vi "fgt set log output mode.vi"(8 "error in (no error)":errorcluster, 9 "output to queue (False)":bool, 10 "output to stderr (False)":bool, 11 "output to file (True)":bool=TRUE) -> (0 "error out":errorcluster)   [LabVIEW 2016, in "fgt_SDK.lvlib"]
doc: "Sets how the SDK outputs the log entries."
uses:
  fgt_SDK.lvlib
  dlls/fgt_SDK_32.dll
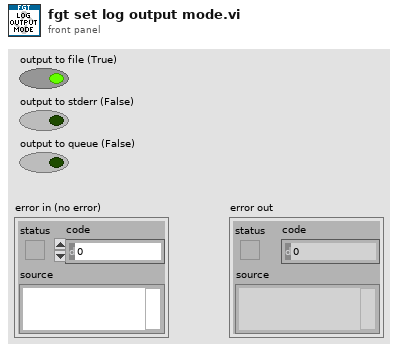
[diagram p1: front panel]
types:
  T1 = typedef "fgt_SDK.lvlib/fgt_STATUS_INFO.ctl" = cluster{"InstrType":T2, "instrSN":u16, "errorCode":u8, "infoCode":u8, "detail":string}
  T2 = typedef "fgt_SDK.lvlib/fgt_INSTRUMENT_TYPE.ctl" = enum32{"None", "MFCS", "MFCS_EZ", "FRP", "LineUP", "IPS", "ESS", "F_OEM", "CFU", "NIFS"}
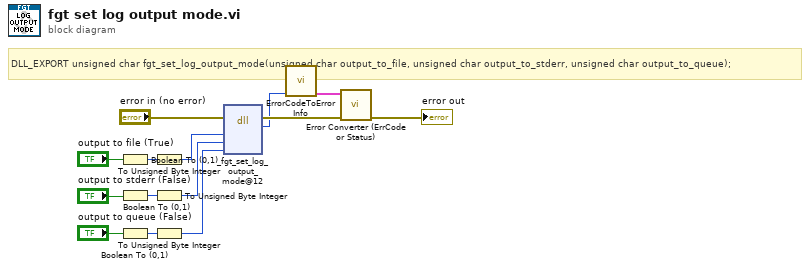
[diagram p0: block diagram]
diagram:
  # "DLL_EXPORT unsigned char fgt_set_log_output_mode(unsigned char output_to_file, unsigned char output_to_stderr, unsigned char output_to_queue);"
  n1 = Boolean To (0,1)(Boolean="output to file (True)") -> (0, 1=w9:i16)
  n2 = Boolean To (0,1)(Boolean="output to stderr (False)") -> (0, 1=w4:i16)
  n3 = Boolean To (0,1)(Boolean="output to queue (False)") -> (0, 1=w3:i16)
  n4 = To Unsigned Byte Integer(number=w9) -> (unsigned 8bit integer=w8:u8)
  n5 = To Unsigned Byte Integer(number=w4) -> (unsigned 8bit integer=w2:u8)
  n6 = To Unsigned Byte Integer(number=w3) -> (unsigned 8bit integer=w1:u8)
  n7 = dll-call lib="C:/projects/SDK/fgt-sdk-labview/dlls/fgt_SDK_*.*" fn="_fgt_set_log_output_mode@12"(error in="error in (no error)", "output to file"=w8, "output to stderr"=w2, "output to queue"=w1) -> (error out=w13:errorcluster, "return type"=w11:u8)  [unwired: 5 in, 1 out]
  n8 = call "ErrorCodeToErrorInfo.vi"("return type"=w11) -> ("StatusInfo"=w10:T1)  [unwired: 10 in]
  n9 = call "Error Converter (ErrCode or Status).vi"("error in (no error)"=w13, "StatusInfo"=w10) -> ("error out"=→"error out":errorcluster)  [unwired: 9 in]
